vi "Celsius To Kelvin.vi"(8 "error in":errorcluster, 11 "Celsius Value":dbl) -> (0 "error out":errorcluster, 3 "Kelvin Value":dbl)   [LabVIEW 2012]
uses:
  <vilib>/ErrorRing/Error Ring.xnode
  <vilib>/Utility/error.llb/Error Cluster From Error Code.vi
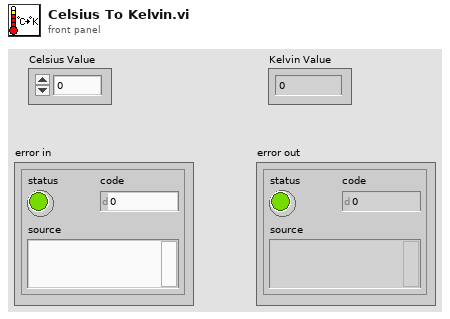
[diagram p1: front panel]
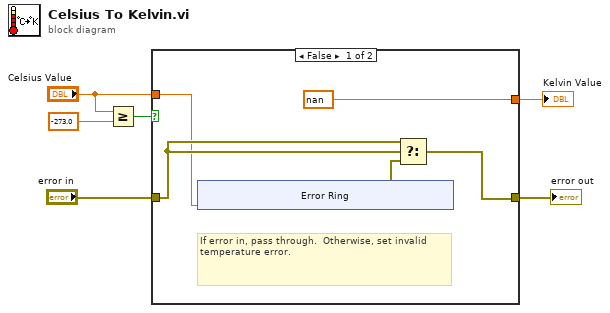
[diagram p0: block diagram]
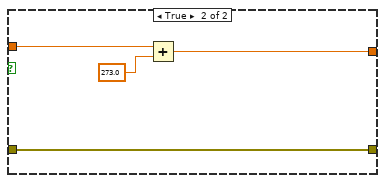
[diagram p2: hidden frame]
diagram:
  n1 = Greater Or Equal?(x="Celsius Value", y=-273.0) -> (x >= y?=w3:bool)
  n2 = case shown="False" w3 {
    tunnel: "Celsius Value" -> [w7 w22]
    tunnel: [nan w21] -> w6
    tunnel: [w9 w19] -> w2
    tunnel: "error in" -> [w10 w19]
    frame False {
      # "If error in, pass through.  Otherwise, set invalid temperature error."
      n3 = xnode "Error Ring"("parameter 0"=w7) -> ("error out"=w8:errorcluster)
      n4 = Select(t=w10, s=w10, f=w8) -> (s? t:f=w9:errorcluster)
    }
    frame True {
      n5 = Add(x=w22, y=273.0) -> (x+y=w21:dbl)
    }
  }
  "Kelvin Value" <- w6
  "error out" <- w2
